vi "Launch Soft Panel.vi"() -> ()   [LabVIEW 2020, in "JMETestSolutions.Instrument.lvlib" / "JMETestSolutions.Instrument.lvclass"]
uses:
  JMETestSolutions.Instrument/JMETestSolutions.Instrument.lvclass
panel:
  in  "Launch Button":bool
  in  "Close Button":bool
  in  "Load Button":bool
  in  "Instrument":string(combo)
  in  "Config File Path":path
  in  "Config":string
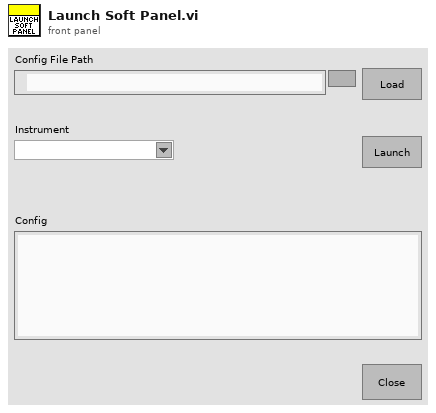
[diagram p1: front panel]
types:
  T1 = typedef "JMETestSolutions.Instrument.lvlib/Named Instrument.ctl" = cluster{"Name":string, "Instrument":refnum<class "JMETestSolutions.Instrument.lvclass">}
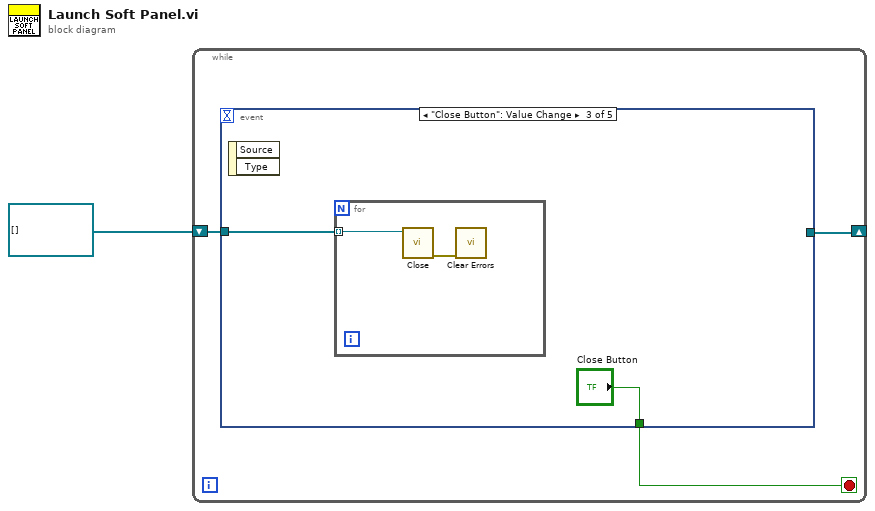
[diagram p0: block diagram]
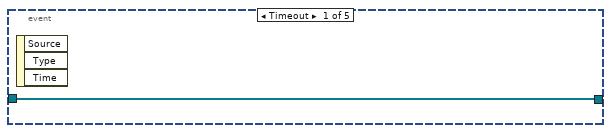
[diagram p2: hidden frame]
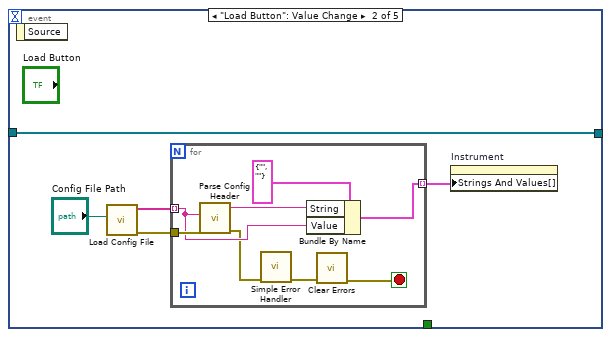
[diagram p3: hidden frame]
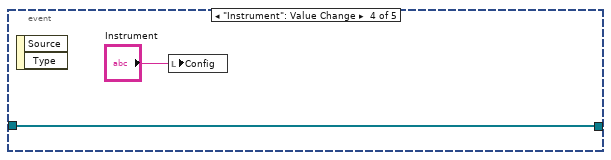
[diagram p4: hidden frame]
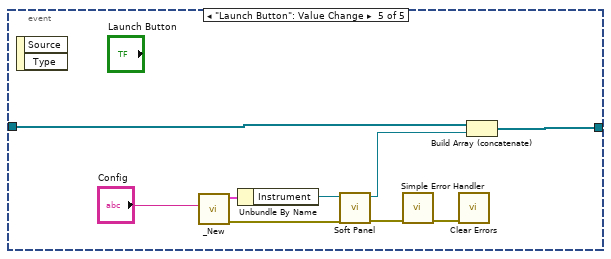
[diagram p5: hidden frame]
diagram:
  n1 = while {
    shift-right: [w2] -> _
    shift-left: refnum<class "JMETestSolutions.Instrument.lvclass">[] [] -> [w3]
    stop <- w4 stop-if-true
    n2 = event shown="[2] \"Close Button\": Value Change" {
      selector: _ -> [_ _ _ _ _]
      dyn-events: _ -> [_ _ _ _ _]
      timeout: _ -> [_ _ _ _ _]
      tunnel: [_ _ "Close Button" _ _] -> w4
      tunnel: w3 -> [w5 w10 w19 w23 w29]
      tunnel: [w5 w10 _ w23 w27] -> w2
      event Timeout {
        n3 = event-data() -> ()  [unwired: 1 in, 3 out]
      }
      event "Load Button": Value Change {
        n4 = event-data() -> ()  [unwired: 1 in, 1 out]
        n5 = call "Load Config File.vi"("Config File Path"="Config File Path") -> ("error out"=w7:errorcluster, "Json Instrument Configurations"=w8:string[])  [unwired: 9 in]
        n6 = for {
          tunnel: w8 -> [w14] mode=indexing
          tunnel: w7 -> [w17]
          tunnel: [w13] -> w6 mode=indexing
          stop <- w12 stop-if-true
          n7 = call "Parse Config Header.vi"("error in (no error)"=w17, "Config String"=w14) -> ("error out"=w11:errorcluster, "name"=w15:string)  [unwired: 6 in, 2 out]
          n8 = call <vilib>:"Simple Error Handler.vi"("error in (no error)"=w11) -> ("error out"=w18:errorcluster)  [unwired: 4 in, 4 out]
          n9 = Bundle By Name(cluster=cluster{"String":string, "Value":string} {"String"="", "Value"=""}, "String"=w15, "Value"=w14) -> (w13:cluster{"String":string, "Value":string})
          n10 = call <vilib>:"Clear Errors.vi"("error in (no error)"=w18) -> ("error out"=w12:errorcluster)  [unwired: 5 in, 1 out]
        }
        n11 = property on="Instrument" class="CmbBox"("Strings And Values[]"=w6) -> ()  [unwired: 2 in, 2 out]
      }
      event "Close Button": Value Change {
        n12 = event-data() -> ()  [unwired: 1 in, 2 out]
        n13 = for {
          tunnel: w19 -> [w22] mode=indexing
          n14 = call-dynamic "Close.vi"("JMETestSolutions.Instrument in"=w22) -> ("error out"=w21:errorcluster)  [unwired: 10 in]
          n15 = call <vilib>:"Clear Errors.vi"("error in (no error)"=w21) -> ()  [unwired: 5 in, 2 out]
        }
      }
      event "Instrument": Value Change {
        n16 = event-data() -> ()  [unwired: 1 in, 2 out]
        n17 = local write "Config"("Instrument") -> ()
      }
      event "Launch Button": Value Change {
        n18 = event-data() -> ()  [unwired: 1 in, 2 out]
        n19 = call "_New.vi"("Configuration"="Config") -> ("error out"=w33:errorcluster, "Instrument"=w31:T1)  [unwired: 9 in]
        n20 = Unbundle By Name(w31) -> ("Instrument"=w32:refnum<class "JMETestSolutions.Instrument.lvclass">)
        n21 = call-dynamic "Soft Panel.vi"("error in (no error)"=w33, "JMETestSolutions.Instrument in"=w32) -> ("error out"=w26:errorcluster, "JMETestSolutions.Instrument out"=w28:refnum<class "JMETestSolutions.Instrument.lvclass">)  [unwired: 8 in]
        n22 = call <vilib>:"Simple Error Handler.vi"("error in (no error)"=w26) -> ("error out"=w25:errorcluster)  [unwired: 4 in, 4 out]
        n23 = call <vilib>:"Clear Errors.vi"("error in (no error)"=w25) -> ()  [unwired: 5 in, 2 out]
        n24 = Build Array (concatenate)(w29, w28) -> (w27:refnum<class "JMETestSolutions.Instrument.lvclass">[])
      }
    }
  }
